vi "Lvi Get Teds Bridge Sensor Info.vi"(7 "HardwareTeds":bool, 8 "error in (no error)":errorcluster, 9 "Channel":u32, 10 "TedsFile":string, 11 "TaskRef":i32) -> (0 "error out":errorcluster, 1 "BridgeSensorTeds":T1, 2 "BasicTeds":T2, 3 "TaskRef out":i32, 5 "function return":i32)   [LabVIEW 2022 SP3, in "DtLvLink.lvlib"]
doc: "Calls directly into the entry points of the DLL of the Data Acq SDK to return TEDS information about a bridge-based sensor."
uses:
  DtLvLink.lvlib
  <userlib>/LV-Link3/DtLvLink_64.dll
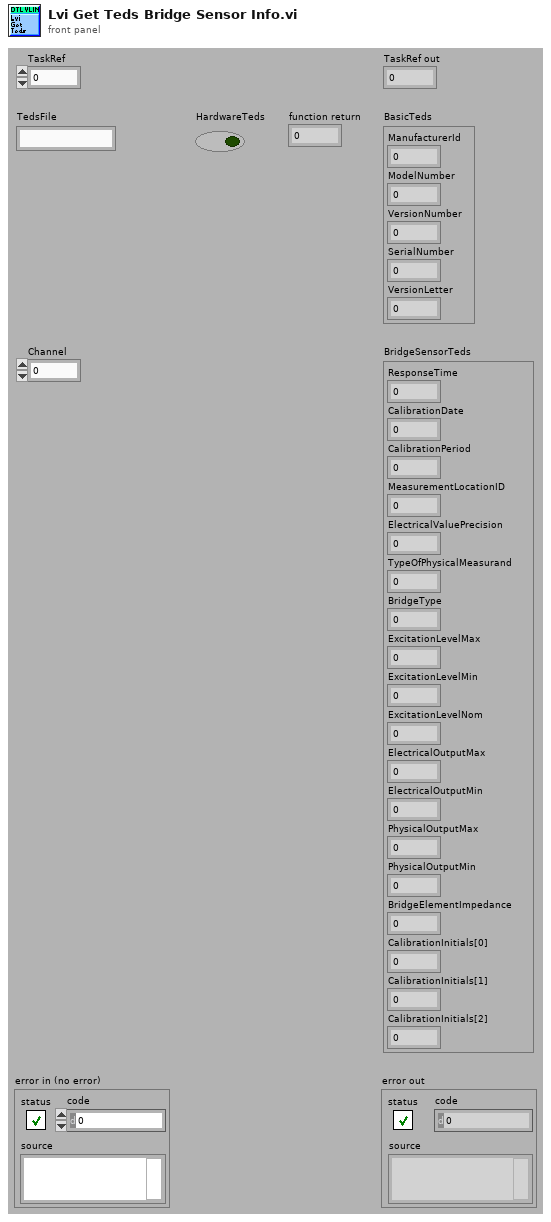
[diagram p1: front panel]
types:
  T1 = cluster{"ResponseTime":dbl, "CalibrationDate":u32, "CalibrationPeriod":u32, "MeasurementLocationID":u32, "ElectricalValuePrecision":u32, "TypeOfPhysicalMeasurand":i32, "BridgeType":i32, "ExcitationLevelMax":sgl, "ExcitationLevelMin":sgl, "ExcitationLevelNom":sgl, "ElectricalOutputMax":sgl, "ElectricalOutputMin":sgl, "PhysicalOutputMax":sgl, "PhysicalOutputMin":sgl, "BridgeElementImpedance":sgl, "CalibrationInitials[0]":i8, "CalibrationInitials[1]":i8, "CalibrationInitials[2]":i8}
  T2 = cluster{"ManufacturerId":i32, "ModelNumber":i32, "VersionNumber":i32, "SerialNumber":u32, "VersionLetter":i8}
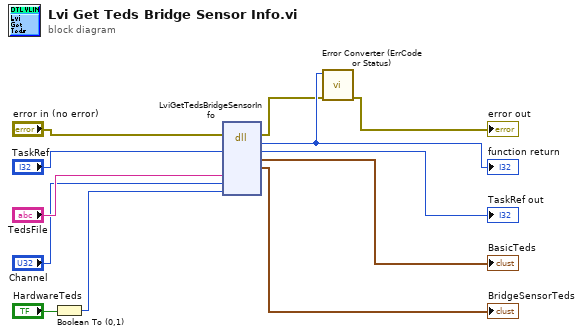
[diagram p0: block diagram]
diagram:
  n1 = Boolean To (0,1)(Boolean="HardwareTeds") -> (0, 1=w4:i16)
  n2 = dll-call lib="C:/Program Files/National Instruments/LabVIEW 2022/user.lib/LV-Link3/DtLvLink_64.*" fn="LviGetTedsBridgeSensorInfo"(error in="error in (no error)", "TaskRef"="TaskRef", "TedsFile"="TedsFile", "Channel"="Channel", "HardwareTeds"=w4) -> (error out=w2:errorcluster, "return type"=w12:i32, "TaskRef"=→"TaskRef out":i32, "BasicTeds"=→"BasicTeds":T2, "BridgeSensorTeds"=→"BridgeSensorTeds":T1)  [unwired: 7 in, 1 out]
  "function return" <- w12
  n3 = call "Error Converter (ErrCode or Status).vi"("error in (no error)"=w2, "error code"=w12) -> ("error out"=→"error out":errorcluster)  [unwired: 9 in]
